vi "PushMany.vi"(10 "Elements":T1[](array[typedef]), 11 "POTTypedCircularBuffer in":refnum<class "POTTypedCircularBuffer.lvclass">) -> (3 "POTTypedCircularBuffer out":refnum<class "POTTypedCircularBuffer.lvclass">)   [LabVIEW 2024, in "POTTypedCircularBuffer.lvclass"]
uses:
  POTTypedCircularBuffer.lvclass
  Type.ctl
  POTTypedCircularBuffer.lvclass/POTTypedCircularBuffer.ctl
  ReadCount.vi
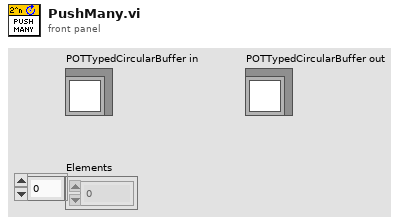
[diagram p1: front panel]
types:
  T1 = typedef "POTTypedCircularBuffer.lvclass/Type.ctl" = i32
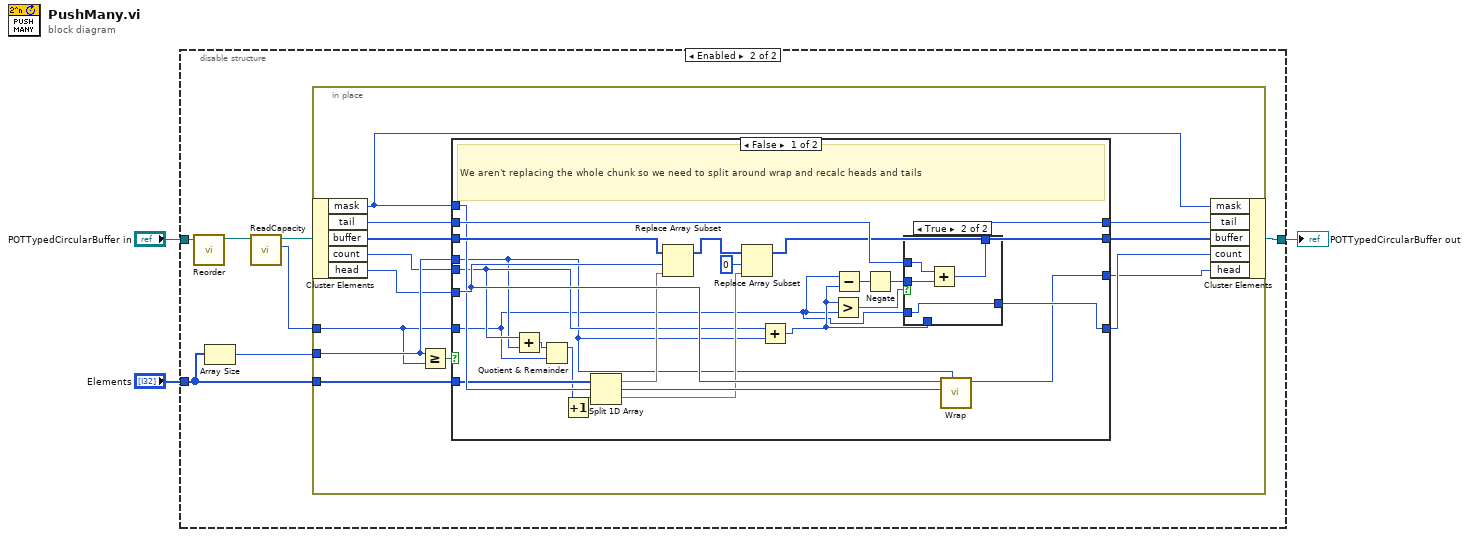
[diagram p0: block diagram]
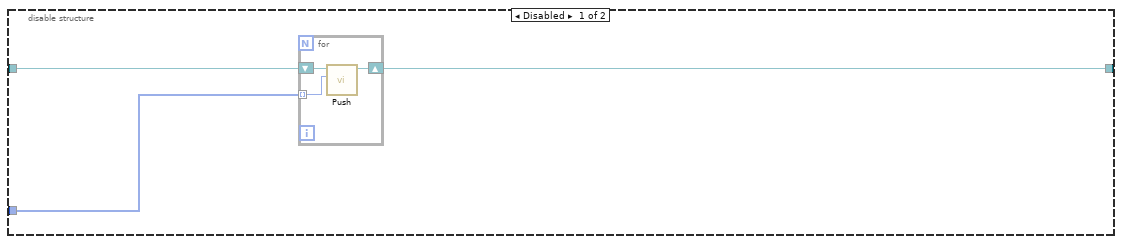
[diagram p2: hidden frame]
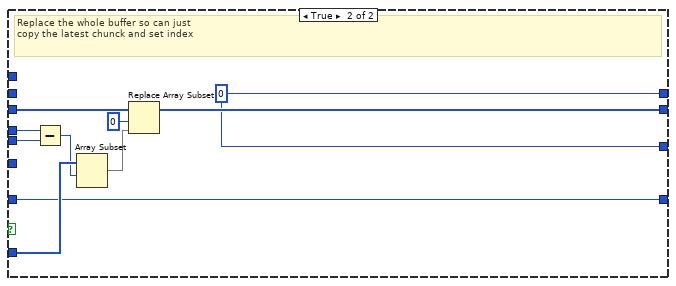
[diagram p4: hidden frame]
diagram:
  n1 = disable-structure shown="Enabled" {
    disable-tunnel: "POTTypedCircularBuffer in" -> [w6 w11]
    disable-tunnel: [w5 w14] -> w2
    disable-tunnel: "Elements" -> [w4 w15]
    frame Disabled {
      n2 = for {
        shift-right: [w8] -> w5
        shift-left: w6 -> [w9]
        tunnel: w4 -> [w7] mode=indexing
        n3 = call "Push.vi"("Element"=w7, "POTTypedCircularBuffer in"=w9) -> ("POTTypedCircularBuffer out"=w8:refnum<class "POTTypedCircularBuffer.lvclass">)  [unwired: 9 in]
      }
    }
    frame Enabled {
      n4 = call "Reorder.vi"("POTTypedCircularBuffer in"=w11) -> ("POTTypedCircularBuffer out"=w10:refnum<class "POTTypedCircularBuffer.lvclass">)  [unwired: 10 in]
      n5 = Array Size(array=w15) -> (size(s)=w16:i32)
      n6 = call "ReadCapacity.vi"("POTTypedCircularBuffer in"=w10) -> ("capacity"=w12:i32, "POTTypedCircularBuffer out"=w13:refnum<class "POTTypedCircularBuffer.lvclass">)  [unwired: 9 in]
      n7 = in-place {
        in-place-border: w16 -> [w25]
        in-place-border: w15 -> [w28]
        in-place-border: w12 -> [w22]
        n8 = in-place-cluster #1(w13) -> ("mask"=w17:i32, "tail"=w19:i32, "buffer"=w29:T1[], "count"=w24:i32, "head"=w21:i32)
        n9 = Greater Or Equal?(x=w25, y=w22) -> (x >= y?=w26:bool)
        n10 = case shown="False" w26 {
          tunnel: w29 -> [w52 w68]
          tunnel: w28 -> [w41 w64]
          tunnel: [w38 w67] -> w27
          tunnel: w25 -> [w34 w66]
          tunnel: w24 -> [w35 w65]
          tunnel: w22 -> [w32 w60]
          tunnel: [w46 w60] -> w23
          tunnel: w21 -> [w43 _]
          tunnel: [w44 w59] -> w20
          tunnel: w19 -> [w49 _]
          tunnel: [w48 w59] -> w18
          tunnel: w17 -> [w42 _]
          frame False {
            # "We aren't replacing the whole chunk so we need to split around wrap and recalc heads and tails"
            n11 = Add(x=w35, y=w34) -> (x+y=w33:i32)
            n12 = Quotient & Remainder(x=w33, y=w32) -> (x-y*floor(x/y)=w31:i32)  [unwired: 1 out]
            n13 = Increment(x=w31) -> (x+1=w30:i32)
            n14 = Split 1D Array(array=w41, index=w30) -> (first subarray=w40:T1[], second subarray=w36:T1[])
            n15 = Replace Array Subset(array=w52, new element=w40, index=w43) -> (w39:T1[])
            n16 = Replace Array Subset(array=w39, new element=w36, index=0) -> (w38:T1[])
            n17 = Add(x=w35, y=w34) -> (x+y=w47:i32)
            n18 = Greater?(x=w47, y=w32) -> (0:w51:bool)
            n19 = Subtract(x=w32, y=w47) -> (x-y=w50:i32)
            n20 = Negate(x=w50) -> (-x=w45:i32)
            n21 = case shown="True" w51 {
              tunnel: w45 -> [_ w58]
              tunnel: w49 -> [w53 w57]
              tunnel: [w53 w56] -> w48
              tunnel: w47 -> [w54 _]
              tunnel: [w54 w55] -> w46
              tunnel: w32 -> [_ w55]
              frame False {
              }
              frame True {
                n22 = Add(x=w57, y=w58) -> (x+y=w56:i32)
              }
            }
            n23 = call "Wrap.vi"("increment amount (1)"=w34, "mask"=w42, "index"=w43) -> ("wrapped"=w44:i32)  [unwired: 8 in]
          }
          frame True {
            w59 = 0 ("tail")
            # "Replace the whole buffer so can just\ncopy the latest chunck and set index"
            n24 = Subtract(x=w66, y=w65) -> (x-y=w63:i32)
            n25 = Array Subset(array=w64, index=w63) -> (w62:T1[])  [unwired: 1 in]
            n26 = Replace Array Subset(array=w68, new element=w62, index=0) -> (w67:T1[])
          }
        }
        n27 = in-place-cluster #1("mask"=w17, "tail"=w18, "buffer"=w27, "count"=w23, "head"=w20) -> (w14:refnum<class "POTTypedCircularBuffer.lvclass">)
      }
    }
  }
  "POTTypedCircularBuffer out" <- w2
